vi "Dynamixel live Position Server.vi"(7 "Theshold":u32=10, 11 "Com port":refnum<visa-resource-name> caption="instrument handle") -> (2 "dynamixel_error":string, 3 "dynamixel_comm_result":string)   [LabVIEW 2022 SP3]
uses:
  Sub Vis/Dynamixel Commands.ctl
  Sub Vis/Dynamixel Global.vi
  Library/dxl.lvlib
panel:
  out "Raw Position":u32
  out "Operating Mode read":u8
  out "Run Time (Sec)":dbl
  out "Waveform Chart":cluster{i32, i32}(graph)
  in  "Terminate Live Position":bool
  out "value : PRO (knob)\npresent position":i32(knob) scale=150000.0..-150000.0
  in  "Max_position_limit_value":u32=4095
  out "port_num":i32
  in  "dynamixel_id":u8=1
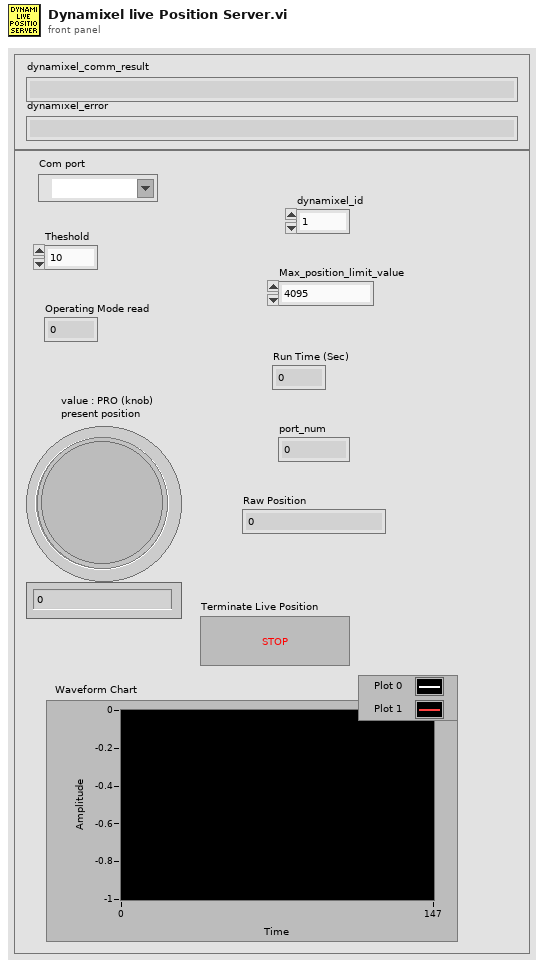
[diagram p1: front panel]
types:
  T1 = typedef "Dynamixel Commands.ctl" = enum16{"Torque Enable", "Present Position", "Threshold", "Max Position Limit", "Acceleration Profile", "Velocity Profile", "Goal Position", "Position Proportional Gain", "Position Integral Gain", "Position Differential Gain ", "Shutdown", "Write Operating Mode", "Read Operating Mode"}
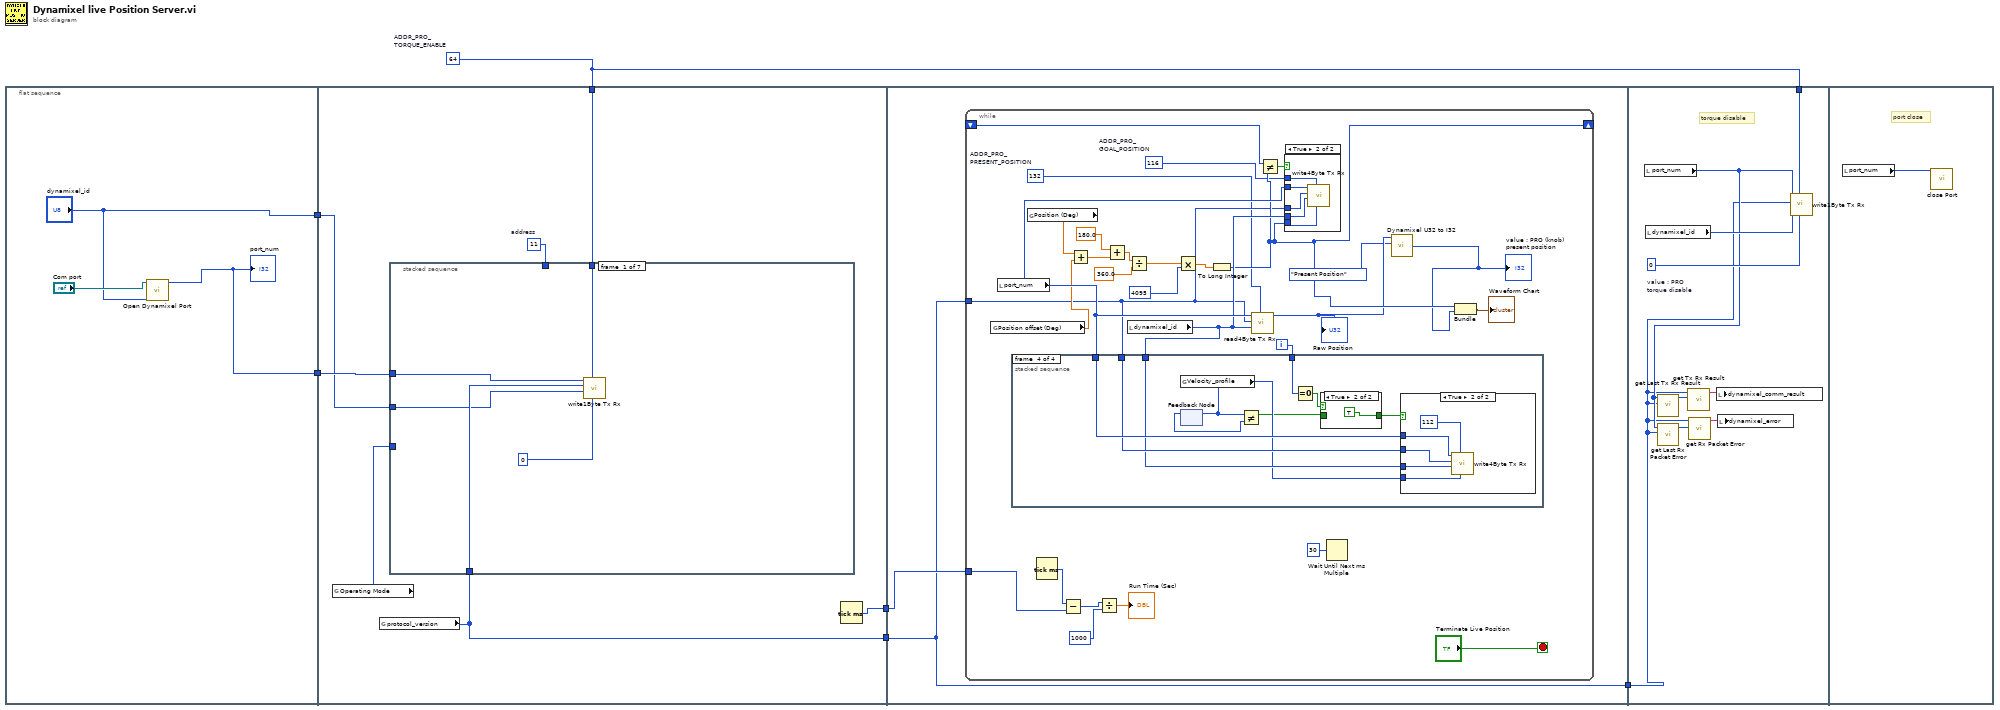
[diagram p0: block diagram]
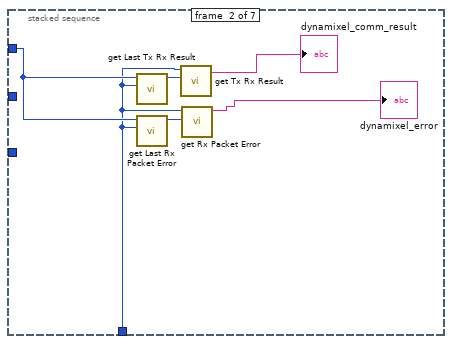
[diagram p2: hidden frame]
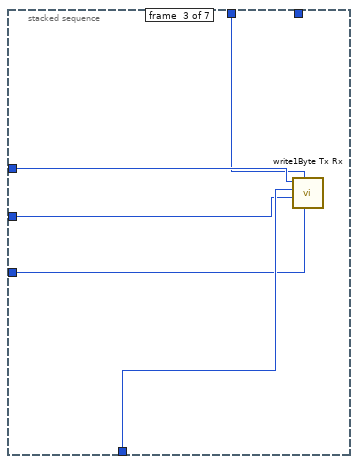
[diagram p3: hidden frame]
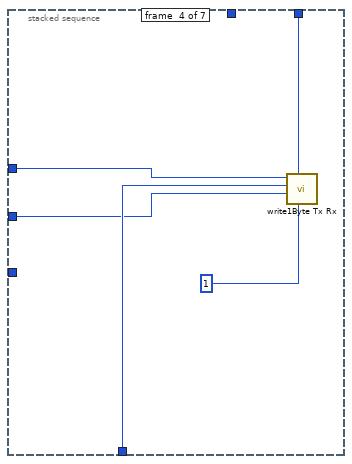
[diagram p4: hidden frame]
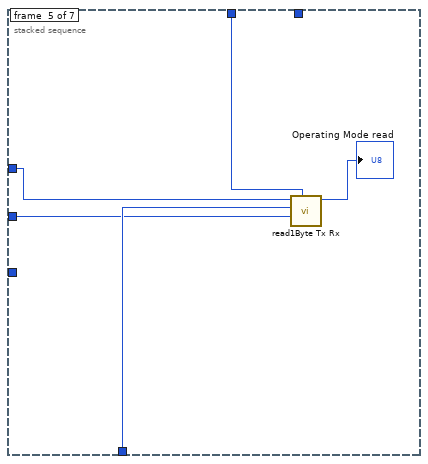
[diagram p5: hidden frame]
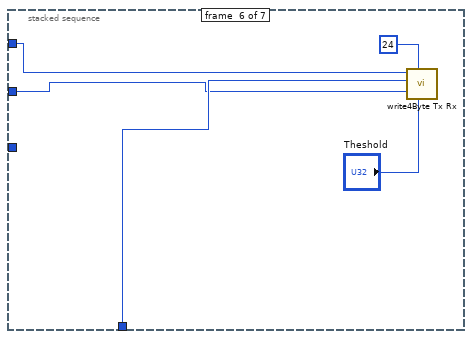
[diagram p6: hidden frame]
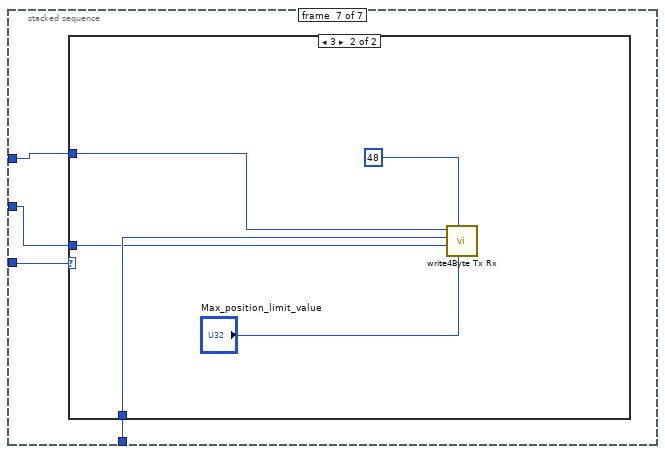
[diagram p7: hidden frame]
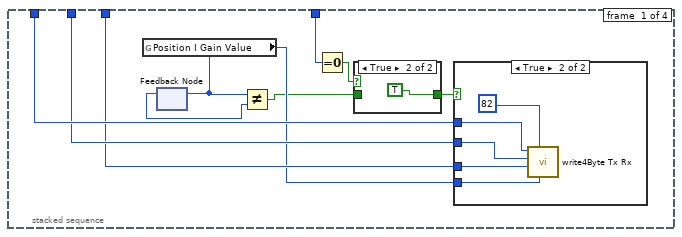
[diagram p9: hidden frame]
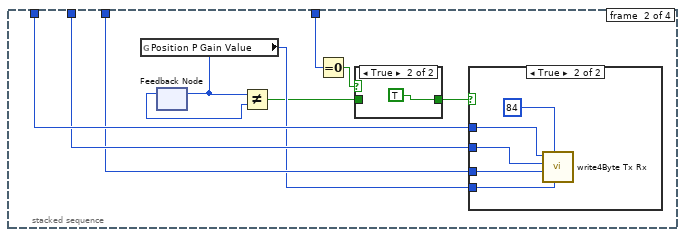
[diagram p12: hidden frame]
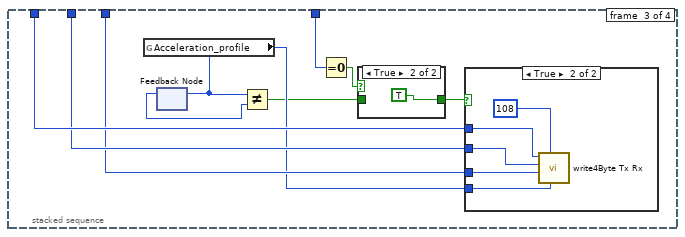
[diagram p15: hidden frame]
diagram:
  w1 = u16 64  # ADDR_PRO_ TORQUE_ENABLE
  n1 = flat-sequence {
    tunnel: ["dynamixel_id"] -> w5
    tunnel: [w7] -> w4
    tunnel: [w16] -> w6
    tunnel: w5 -> [w14]
    tunnel: w4 -> [w15]
    tunnel: [w12] -> w3
    tunnel: w1 -> [w10]
    tunnel: w6 -> [w58]
    tunnel: w3 -> [w57]
    tunnel: [w57] -> w2
    tunnel: w2 -> [w158]
    tunnel: w1 -> [w157]
    frame #0 {
      n2 = call "Open Dynamixel Port.vi"("dynamixel_id"="dynamixel_id", "Com port"="Com port") -> ("port_num"=w7:i32)  [unwired: 7 in, 2 out]
      "port_num" <- w7
    }
    frame #1 {
      w13 = u16 11  # address
      n3 = global read "Dynamixel Global.vi" "Operating Mode"() -> (w11:u8)
      n4 = global read "Dynamixel Global.vi" "protocol_version"() -> (w12:i32)
      n5 = stacked-sequence {
        tunnel: w15 -> [w21 w23 w32 w37 w40 w46 w50]
        tunnel: w10 -> [w20 _ _ w36 _ _ _]
        tunnel: w12 -> [w19 w22 w31 w35 w39 w45 w49]
        tunnel: w14 -> [w18 _ w30 w34 w38 w44 w48]
        tunnel: w13 -> [_ _ w29 _ w41 _ _]
        tunnel: w11 -> [_ _ w28 _ _ _ w51]
        frame #0 {
          n6 = call "write1Byte Tx Rx.vi"("data"=u8 0, "address"=w20, "id"=w18, "protocol_version"=w19, "port_num"=w21) -> ()  [unwired: 6 in, 1 out]
        }
        frame #1 {
          n7 = call "get Last Tx Rx Result.vi"("protocol_version"=w22, "port_num"=w23) -> ("function return"=w27:i32)  [unwired: 8 in, 1 out]
          n8 = call "get Last Rx Packet Error.vi"("protocol_version"=w22, "port_num"=w23) -> ("function return"=w26:u8)  [unwired: 8 in, 1 out]
          n9 = call "get Tx Rx Result.vi"("result"=w27, "protocol_version"=w22) -> ("function return"=→"dynamixel_comm_result":string)  [unwired: 8 in, 1 out]
          n10 = call "get Rx Packet Error.vi"("error"=w26, "protocol_version"=w22) -> ("function return"=→"dynamixel_error":string)  [unwired: 8 in, 1 out]
        }
        frame #2 {
          n11 = call "write1Byte Tx Rx.vi"("data"=w28, "address"=w29, "id"=w30, "protocol_version"=w31, "port_num"=w32) -> ()  [unwired: 6 in, 1 out]
        }
        frame #3 {
          n12 = call "write1Byte Tx Rx.vi"("data"=u8 1, "address"=w36, "id"=w34, "protocol_version"=w35, "port_num"=w37) -> ()  [unwired: 6 in, 1 out]
        }
        frame #4 {
          n13 = call "read1Byte Tx Rx.vi"("address"=w41, "id"=w38, "protocol_version"=w39, "port_num"=w40) -> ("function return"=→"Operating Mode read":u8)  [unwired: 6 in, 1 out]
        }
        frame #5 {
          n14 = call "write4Byte Tx Rx.vi"("data"="Theshold", "address"=u16 24 ("ADDR_Theshold"), "id"=w44, "protocol_version"=w45, "port_num"=w46) -> ()  [unwired: 6 in, 1 out]
        }
        frame #6 {
          n15 = case shown="3" w51 {
            tunnel: w50 -> [_ w55]
            tunnel: w49 -> [_ w54]
            tunnel: w48 -> [_ w53]
            frame 0, Default {
            }
            frame 3 {
              n16 = call "write4Byte Tx Rx.vi"("data"="Max_position_limit_value", "address"=u16 48 ("ADDR_Max_Position_Limit"), "id"=w53, "protocol_version"=w54, "port_num"=w55) -> ()  [unwired: 6 in, 1 out]
            }
          }
        }
      }
      n17 = Tick Count (ms)() -> (millisecond timer value=w16:u32)
    }
    frame #2 {
      n18 = while {
        tunnel: w58 -> [w80]
        shift-right: [w69] -> _
        shift-left: _ -> [w85]
        tunnel: w57 -> [w64]
        i -> [w76]
        stop <- "Terminate Live Position" stop-if-true
        w62 = u16 116  # ADDR_PRO_ GOAL_POSITION
        w63 = u16 132  # ADDR_PRO_ PRESENT_POSITION
        n19 = global read "Dynamixel Global.vi" "Position offset (Deg)"() -> (w74:dbl)
        n20 = local read "port_num"() -> (w83:i32)
        n21 = global read "Dynamixel Global.vi" "Position (Deg)"() -> (w75:dbl)
        n22 = Tick Count (ms)() -> (millisecond timer value=w81:u32)
        n23 = Subtract(x=w81, y=w80) -> (x-y=w79:u32)
        n24 = Add(x=w75, y=w74) -> (x+y=w61:dbl)
        n25 = Divide(x=w79, y=u32 1000) -> (x/y=→"Run Time (Sec)":dbl)
        n26 = Add(x=180.0, y=w61) -> (x+y=w59:dbl)
        n27 = local read "dynamixel_id"() -> (w82:u8)
        n28 = stacked-sequence {
          tunnel: w83 -> [w96 w112 w128 w144]
          tunnel: w64 -> [w95 w111 w127 w143]
          tunnel: w82 -> [w94 w110 w126 w142]
          tunnel: w76 -> [w91 w104 w120 w138]
          frame #0 {
            n29 = global read "Dynamixel Global.vi" "Position I Gain Value"() -> (w93:u32)
            n30 = feedback-in #1(w93) -> ()
            n31 = feedback #1() -> (w92:u32)  [unwired: 1 in]
            n32 = Not Equal?(x=w93, y=w92) -> (x != y?=w89:bool)
            n33 = Equal To 0?(x=w91) -> (x = 0?=w90:bool)
            n34 = case shown="True" w90 {
              tunnel: [w97 TRUE] -> w88
              tunnel: w89 -> [w97 _]
              frame False {
              }
              frame True {
              }
            }
            n35 = case shown="True" w88 {
              tunnel: w96 -> [_ w103]
              tunnel: w95 -> [_ w102]
              tunnel: w94 -> [_ w101]
              tunnel: w93 -> [_ w100]
              frame False {
              }
              frame True {
                n36 = call "write4Byte Tx Rx.vi"("data"=w100, "address"=u16 82 ("ADDR_Position_I_Gain"), "id"=w101, "protocol_version"=w102, "port_num"=w103) -> ()  [unwired: 6 in, 1 out]
              }
            }
          }
          frame #1 {
            n37 = global read "Dynamixel Global.vi" "Position P Gain Value"() -> (w109:u32)
            n38 = feedback-in #2(w109) -> ()
            n39 = feedback #2() -> (w108:u32)  [unwired: 1 in]
            n40 = Not Equal?(x=w109, y=w108) -> (x != y?=w106:bool)
            n41 = Equal To 0?(x=w104) -> (x = 0?=w107:bool)
            n42 = case shown="True" w107 {
              tunnel: [w113 TRUE] -> w105
              tunnel: w106 -> [w113 _]
              frame False {
              }
              frame True {
              }
            }
            n43 = case shown="True" w105 {
              tunnel: w112 -> [_ w119]
              tunnel: w111 -> [_ w118]
              tunnel: w110 -> [_ w117]
              tunnel: w109 -> [_ w116]
              frame False {
              }
              frame True {
                n44 = call "write4Byte Tx Rx.vi"("data"=w116, "address"=u16 84, "id"=w117, "protocol_version"=w118, "port_num"=w119) -> ()  [unwired: 6 in, 1 out]
              }
            }
          }
          frame #2 {
            n45 = global read "Dynamixel Global.vi" "Acceleration_profile"() -> (w125:u32)
            n46 = feedback-in #3(w125) -> ()
            n47 = feedback #3() -> (w124:u32)  [unwired: 1 in]
            n48 = Not Equal?(x=w125, y=w124) -> (x != y?=w122:bool)
            n49 = Equal To 0?(x=w120) -> (x = 0?=w123:bool)
            n50 = case shown="True" w123 {
              tunnel: [w129 TRUE] -> w121
              tunnel: w122 -> [w129 _]
              frame False {
              }
              frame True {
              }
            }
            n51 = case shown="True" w121 {
              tunnel: w128 -> [_ w135]
              tunnel: w127 -> [_ w134]
              tunnel: w126 -> [_ w133]
              tunnel: w125 -> [_ w132]
              frame False {
              }
              frame True {
                n52 = call "write4Byte Tx Rx.vi"("data"=w132, "address"=u16 108, "id"=w133, "protocol_version"=w134, "port_num"=w135) -> ()  [unwired: 6 in, 1 out]
              }
            }
          }
          frame #3 {
            n53 = global read "Dynamixel Global.vi" "Velocity_profile"() -> (w141:u32)
            n54 = feedback-in #4(w141) -> ()
            n55 = feedback #4() -> (w140:u32)  [unwired: 1 in]
            n56 = Not Equal?(x=w141, y=w140) -> (x != y?=w137:bool)
            n57 = Equal To 0?(x=w138) -> (x = 0?=w139:bool)
            n58 = case shown="True" w139 {
              tunnel: [w145 TRUE] -> w136
              tunnel: w137 -> [w145 _]
              frame False {
              }
              frame True {
              }
            }
            n59 = case shown="True" w136 {
              tunnel: w144 -> [_ w151]
              tunnel: w143 -> [_ w150]
              tunnel: w142 -> [_ w149]
              tunnel: w141 -> [_ w148]
              frame False {
              }
              frame True {
                n60 = call "write4Byte Tx Rx.vi"("data"=w148, "address"=u16 112, "id"=w149, "protocol_version"=w150, "port_num"=w151) -> ()  [unwired: 6 in, 1 out]
              }
            }
          }
        }
        n61 = Divide(x=w59, y=360.0) -> (x/y=w68:dbl)
        n62 = Multiply(x=w68, y=4095) -> (x*y=w70:dbl)
        n63 = To Long Integer(number=w70) -> (32bit integer=w69:i32)
        n64 = call "read4Byte Tx Rx.vi"("address"=w63, "id"=w82, "protocol_version"=w64, "port_num"=w83) -> ("function return"=w67:u32)  [unwired: 6 in, 1 out]
        "Raw Position" <- w67
        n65 = Not Equal?(x=w85, y=w69) -> (x != y?=w86:bool)
        n66 = case shown="True" w86 {
          tunnel: w62 -> [_ w156]
          tunnel: w83 -> [_ w155]
          tunnel: w64 -> [_ w154]
          tunnel: w82 -> [_ w153]
          tunnel: w69 -> [_ w152]
          frame False {
          }
          frame True {
            n67 = call "write4Byte Tx Rx.vi"("data"=w152, "address"=w156, "id"=w153, "protocol_version"=w154, "port_num"=w155) -> ()  [unwired: 6 in, 1 out]
          }
        }
        n68 = Wait Until Next ms Multiple(millisecond multiple=u32 30) -> ()  [unwired: 1 out]
        n69 = call "Dynamixel U32 to I32.vi"("U32 In"=w67, "Function"=Dynamixel_Commands."Present Position") -> ("I32 Out"=w65:i32)  [unwired: 3 in]
        "value : PRO (knob)\npresent position" <- w65
        n70 = Bundle(w69, "I32 Out"=w65) -> (→"Waveform Chart":cluster{i32, "I32 Out":i32})  [unwired: 1 in]
      }
    }
    frame #3 {
      w164 = 0  # value : PRO torque disable
      # "torque disable"
      n71 = local read "port_num"() -> (w161:i32)
      n72 = local read "dynamixel_id"() -> (w165:u8)
      n73 = call "get Last Tx Rx Result.vi"("protocol_version"=w158, "port_num"=w161) -> ("function return"=w162:i32)  [unwired: 8 in, 1 out]
      n74 = call "get Last Rx Packet Error.vi"("protocol_version"=w158, "port_num"=w161) -> ("function return"=w163:u8)  [unwired: 8 in, 1 out]
      n75 = call "get Tx Rx Result.vi"("result"=w162, "protocol_version"=w158) -> ("function return"=w160:string)  [unwired: 8 in, 1 out]
      n76 = call "get Rx Packet Error.vi"("error"=w163, "protocol_version"=w158) -> ("function return"=w159:string)  [unwired: 8 in, 1 out]
      n77 = local write "dynamixel_comm_result"(w160) -> ()
      n78 = local write "dynamixel_error"(w159) -> ()
      n79 = call "write1Byte Tx Rx.vi"("data"=w164, "address"=w157, "id"=w165, "protocol_version"=w158, "port_num"=w161) -> ()  [unwired: 6 in, 1 out]
    }
    frame #4 {
      # "port close"
      n80 = local read "port_num"() -> (w166:i32)
      n81 = call "close Port.vi"("port_num"=w166) -> ()  [unwired: 10 in, 1 out]
    }
  }
